vi "Test Serialize Special Numbers.vi"(8 "error in (no error)":errorcluster) -> (0 "error out":errorcluster)   [LabVIEW 2013]
uses:
  src/Serializer/JSON Serializer/JSON Serializer.lvclass
  <vilib>/addons/_JKI Toolkits/Caraya/classes/Test/Test.lvclass
  <vilib>/addons/_JKI Toolkits/Caraya/classes/Assert/Assert.lvclass
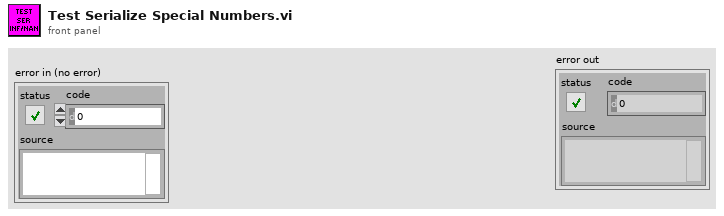
[diagram p1: front panel]
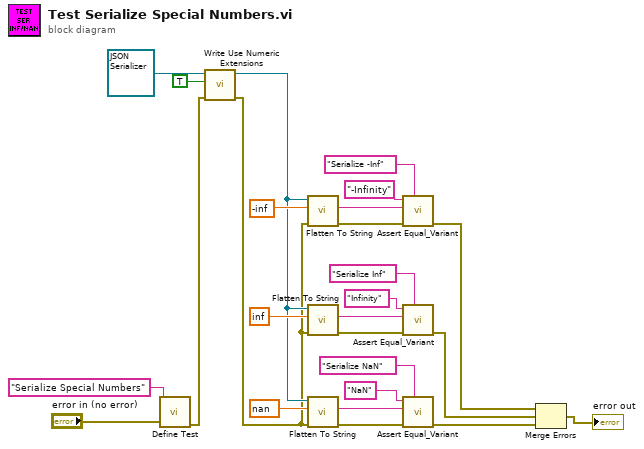
[diagram p0: block diagram]
diagram:
  n1 = call <vilib>:"Define Test.vi"("error in (no error)"="error in (no error)", "Label (VI Title)"="Serialize Special Numbers") -> ("error out"=w2:errorcluster)  [unwired: 9 in]
  n2 = call-dynamic "Write Use Numeric Extensions.vi"("error in (no error)"=w2, "Numeric Extensions"=TRUE, "JSON Serializer in"=refnum<class "JSON Serializer.lvclass"> refnum ("JKI JSON Serialization.lvlib:JSON Serializer.lvclass")) -> ("error out"=w1:errorcluster, "JSON Serializer out"=w4:refnum<class "JSON Serializer.lvclass">)  [unwired: 7 in]
  n3 = call-dynamic "Flatten To String.vi"("error in (no error)"=w1, "Variant"=-inf, "JSON Serializer in"=w4) -> ("error out"=w16:errorcluster, "String"=w15:string)  [unwired: 6 in, 1 out]
  n4 = call-dynamic "Flatten To String.vi"("error in (no error)"=w1, "Variant"=inf, "JSON Serializer in"=w4) -> ("error out"=w20:errorcluster, "String"=w19:string)  [unwired: 6 in, 1 out]
  n5 = call-dynamic "Flatten To String.vi"("error in (no error)"=w1, "Variant"=nan, "JSON Serializer in"=w4) -> ("error out"=w24:errorcluster, "String"=w23:string)  [unwired: 6 in, 1 out]
  n6 = call <vilib>:"Assert Equal_Variant.vi"("Label"="Serialize -Inf", "error in (no error)"=w16, "Y"=w15, "X"="-Infinity") -> ("error out"=w8:errorcluster)  [unwired: 7 in]
  n7 = call <vilib>:"Assert Equal_Variant.vi"("Label"="Serialize Inf", "error in (no error)"=w20, "Y"=w19, "X"="Infinity") -> ("error out"=w9:errorcluster)  [unwired: 7 in]
  n8 = call <vilib>:"Assert Equal_Variant.vi"("Label"="Serialize NaN", "error in (no error)"=w24, "Y"=w23, "X"="NaN") -> ("error out"=w10:errorcluster)  [unwired: 7 in]
  n9 = Merge Errors(w8, w9, w10) -> (→"error out":errorcluster)
